vi "Main.vi"(0 "A":dbl=4.0 min=0.0, 5 "B":dbl=2.0, 7 "Calculate":bool, 11 "Error In":errorcluster, 13 "Operation":T1) -> (4 "Output":dbl=6.0, 15 "error out":errorcluster)   [LabVIEW 2021, in "Calculator.lvlib"]
doc: "This VI acts as a simple calculator using OOPS . There are four seperate child classes for each arithmetic operation which has its overriding method operation.vi . The user selects the operation to perform and gives the input. The output is displayed when calculate is pressed."
uses:
  Calculator.lvlib
  Controls/QueueOperations.ctl
  Controls/Operation.ctl
  Controls/DataCluster.ctl
  Classes/NumericOperation/NumericOperation.lvclass
panel:
  in  "Instruction":bool
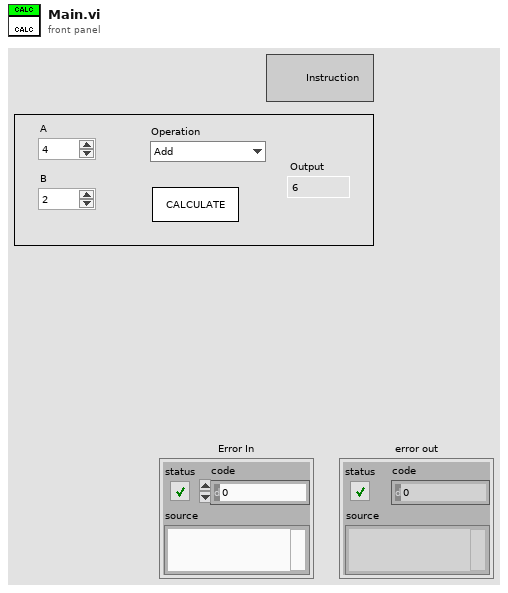
[diagram p1: front panel]
types:
  T1 = typedef "Calculator.lvlib/Operation.ctl" = enum16{"Add", "Subtract", "Multiply", "Divide"}
  T2 = typedef "Calculator.lvlib/QueueOperations.ctl" = enum16{"Create", "Enqueue", "EnqueueN", "Enqueue at Top", "Dequeue", "Flush", "Release"}
  T3 = typedef "Calculator.lvlib/DataCluster.ctl" = cluster{"A":dbl, "B":dbl, "C":dbl, "Operation":T1, "NumericOperation.lvclass":refnum<class "NumericOperation.lvclass">, "generic class reference":refnum<class "NumericOperation.lvclass">, "Base Path":path}
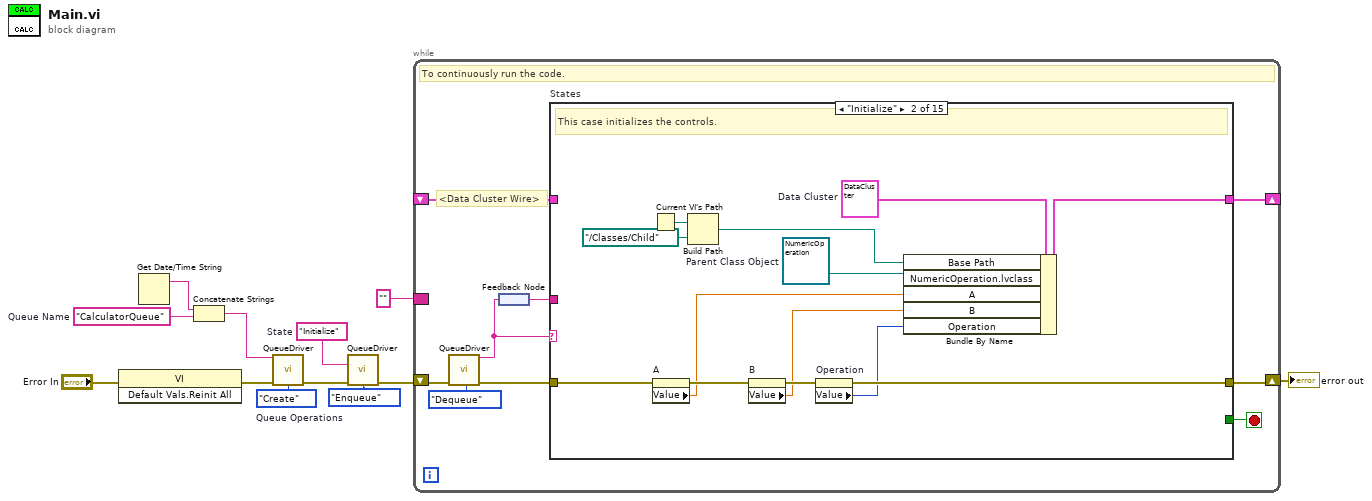
[diagram p0: block diagram]
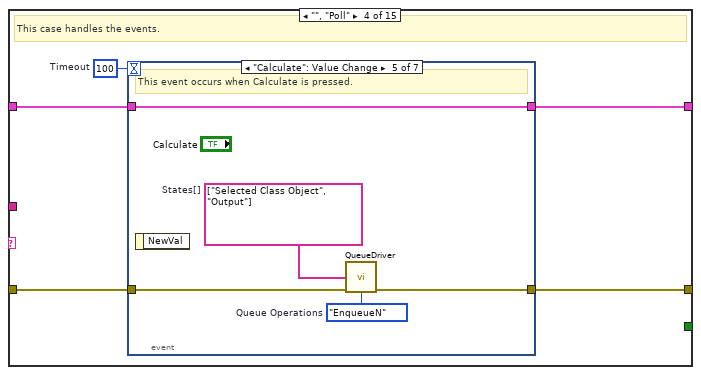
[diagram p4: hidden frame]
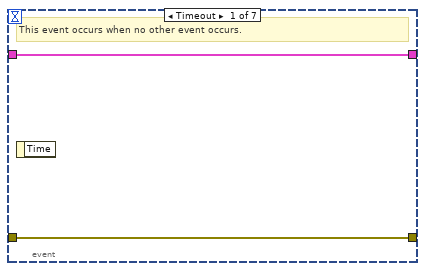
[diagram p5: hidden frame]
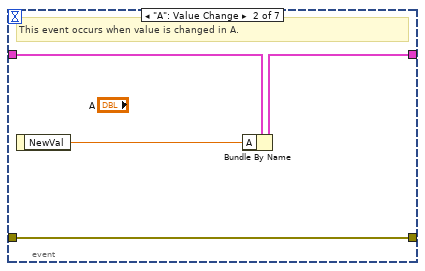
[diagram p6: hidden frame]
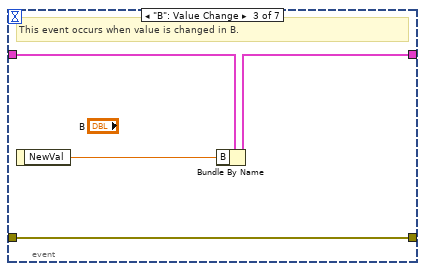
[diagram p7: hidden frame]
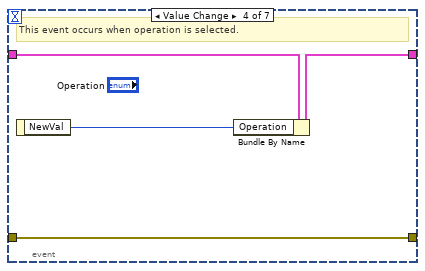
[diagram p8: hidden frame]
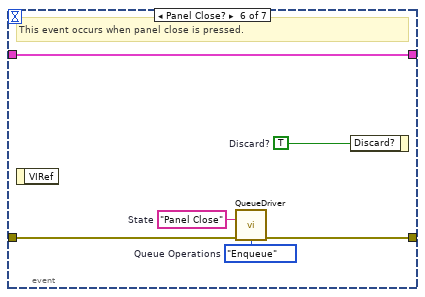
[diagram p9: hidden frame]
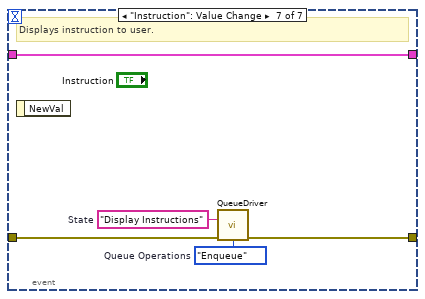
[diagram p10: hidden frame]
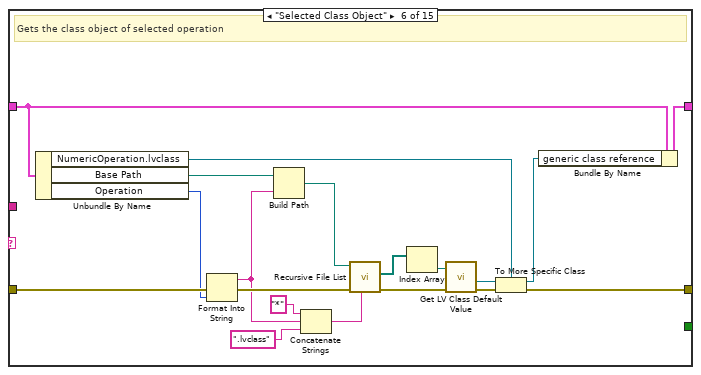
[diagram p12: hidden frame]
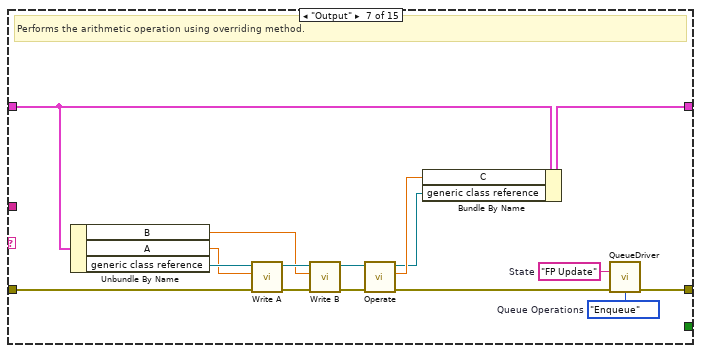
[diagram p13: hidden frame]
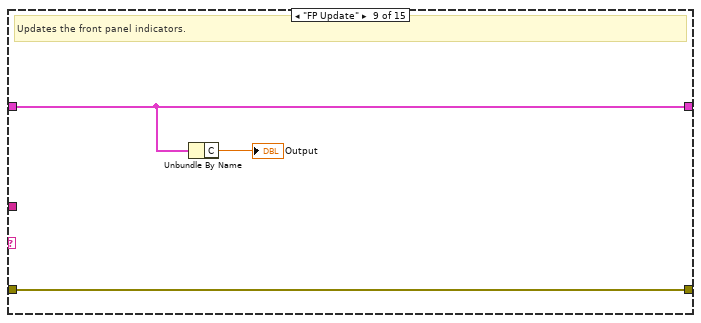
[diagram p15: hidden frame]
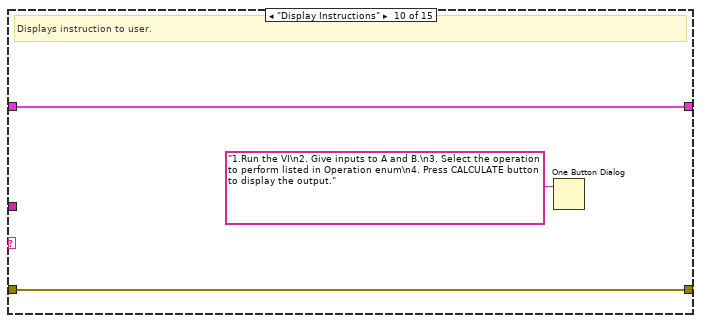
[diagram p16: hidden frame]
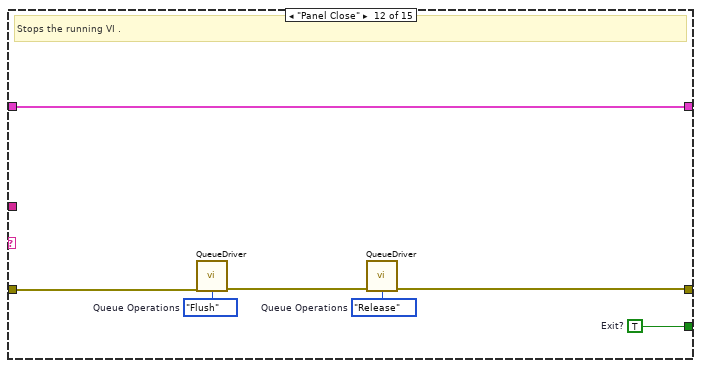
[diagram p18: hidden frame]
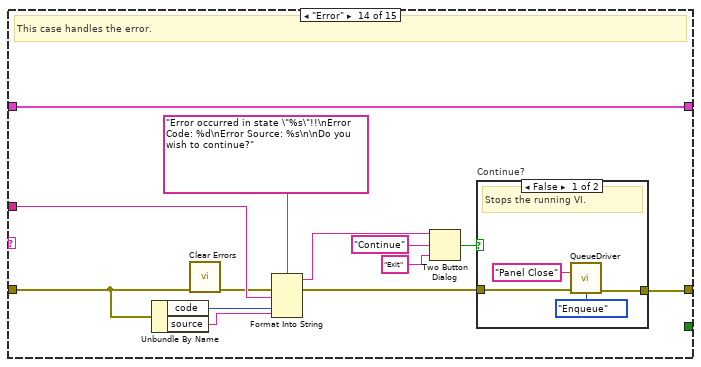
[diagram p20: hidden frame]
diagram:
  w8 = "Initialize"  # State
  w4 = "CalculatorQueue"  # Queue Name
  w11 = QueueOperations."Create"  # Queue Operations
  n1 = invoke class="VI" method="Default Vals.Reinit All"(error in="Error In") -> (error out=w1:errorcluster)  [unwired: 2 in, 2 out]
  n2 = Get Date/Time String() -> (date string=w5:string)  [unwired: 3 in, 1 out]
  n3 = Concatenate Strings(w5, w4) -> (w3:string)
  n4 = call "QueueDriver.vi"("Queue Name"=w3, "Error In"=w1, "Queue Operations"=w11) -> ("Error Out"=w10:errorcluster)  [unwired: 11 in, 1 out]
  n5 = call "QueueDriver.vi"("State"=w8, "Error In"=w10, "Queue Operations"=QueueOperations."Enqueue") -> ("Error Out"=w7:errorcluster)  [unwired: 11 in, 1 out]
  n6 = while {
    shift-right: [w19] -> _
    shift-left: _ -> [w20]
    shift-right: [w17] -> w12
    shift-left: w7 -> [w18]
    border: "" ("Dequeued Element") -> [_]
    stop <- w14 stop-if-true
    # "<Data Cluster Wire>"
    # "To continuously run the code."
    n7 = call "QueueDriver.vi"("Error In"=w18, "Queue Operations"=QueueOperations."Dequeue") -> ("Dequeued Element"=w16:string, "Error Out"=w13:errorcluster)  [unwired: 12 in]
    n8 = feedback-in #1(w16) -> ()
    n9 = feedback #1() -> (w15:string)
    n10 = case "States" shown="\"Initialize\"" w16 {
      tunnel: w20 -> [w23 _ w38 w42 w75 w78 w110 w112 w114 w118 w120 w123 w129 w134 w149]
      tunnel: [w23 w35 w38 w41 w75 w77 w108 w112 w114 w118 w120 w123 w129 w134 w149] -> w19
      tunnel: [w22 w31 w37 w40 w74 w81 w106 w111 w113 w117 w119 w124 w128 w136 w148] -> w17
      tunnel: w15 -> [_ _ _ _ _ _ _ _ _ _ _ _ _ w141 _]
      tunnel: [_ _ _ _ _ _ _ _ _ _ _ w122 _ _ _] -> w14
      tunnel: w13 -> [w22 w34 w37 w39 w74 w94 w96 w111 w113 w117 w119 w121 w128 w131 w148]
      frame "/******** Initialize********/" {
        # "Splitter case for initialization."
      }
      frame "Initialize" {
        w27 = T3 {"A"=0.0, "B"=0.0, "C"=0.0, "Operation"=enum."Add", "NumericOperation.lvclass"=refnum, "generic class reference"=refnum, "Base Path"=path ""}  # Data Cluster
        w36 = refnum<class "NumericOperation.lvclass"> refnum  # Parent Class Object
        # "This case initializes the controls."
        n11 = Current VI's Path() -> (path=w26:path)
        n12 = property on="A" class="DigNum (strict)"(error in=w34) -> (error out=w33:errorcluster, "Value"=w28:dbl)  [unwired: 1 in, 1 out]
        n13 = Build Path(base path=w26, name or relative path=path "../Classes/Child") -> (appended path=w24:path)
        n14 = property on="B" class="DigNum (strict)"(error in=w33) -> (error out=w32:errorcluster, "Value"=w29:dbl)  [unwired: 1 in, 1 out]
        n15 = property on="Operation" class="Enum (strict)"(error in=w32) -> (error out=w31:errorcluster, "Value"=w30:T1)  [unwired: 1 in, 1 out]
        n16 = Bundle By Name(cluster=w27, "Base Path"=w24, "NumericOperation.lvclass"=w36, "A"=w28, "B"=w29, "Operation"=w30) -> (w35:T3)
      }
      frame "/******** Poll ********/" {
        # "Splitter case for poll."
      }
      frame "", "Poll" {
        w43 = 100  # Timeout
        # "This case handles the events."
        n17 = event shown="[4] \"Calculate\": Value Change" {
          selector: _ -> [_ _ _ _ _ _ _]
          dyn-events: _ -> [_ _ _ _ _ _ _]
          timeout: w43 -> [_ _ _ _ _ _ _]
          tunnel: w42 -> [w45 w49 w53 w57 w62 w65 w69]
          tunnel: [w45 w47 w51 w55 w62 w65 w69] -> w41
          tunnel: [w44 w46 w50 w54 w60 w67 w72] -> w40
          tunnel: w39 -> [w44 w46 w50 w54 w61 w63 w73]
          event Timeout {
            # "This event occurs when no other event occurs."
            n18 = event-data() -> ()  [unwired: 1 in, 1 out]
          }
          event "A": Value Change {
            # "This event occurs when value is changed in A."
            n19 = event-data() -> ("NewVal"=w48:dbl)  [unwired: 1 in]
            n20 = Bundle By Name(cluster=w49, "A"=w48) -> (w47:T3)
          }
          event "B": Value Change {
            # "This event occurs when value is changed in B."
            n21 = event-data() -> ("NewVal"=w52:dbl)  [unwired: 1 in]
            n22 = Bundle By Name(cluster=w53, "B"=w52) -> (w51:T3)
          }
          event Value Change {
            # "This event occurs when operation is selected."
            n23 = event-data() -> ("NewVal"=w56:T1)  [unwired: 1 in]
            n24 = Bundle By Name(cluster=w57, "Operation"=w56) -> (w55:T3)
          }
          event "Calculate": Value Change {
            w58 = string[] ["Selected Class Object", "Output"]  # States[]
            w59 = QueueOperations."EnqueueN"  # Queue Operations
            # "This event occurs when Calculate is pressed."
            n25 = event-data() -> ()  [unwired: 1 in, 1 out]
            n26 = call "QueueDriver.vi"("States[]"=w58, "Error In"=w61, "Queue Operations"=w59) -> ("Error Out"=w60:errorcluster)  [unwired: 11 in, 1 out]
          }
          event Panel Close? {
            w64 = QueueOperations."Enqueue"  # Queue Operations
            w66 = "Panel Close"  # State
            w68 = TRUE  # Discard?
            # "This event occurs when panel close is pressed."
            n27 = event-data() -> ()  [unwired: 1 in, 1 out]
            n28 = call "QueueDriver.vi"("State"=w66, "Error In"=w63, "Queue Operations"=w64) -> ("Error Out"=w67:errorcluster)  [unwired: 11 in, 1 out]
            n29 = event-data("Discard?"=w68) -> ()  [unwired: 1 in, 1 out]
          }
          event "Instruction": Value Change {
            w70 = "Display Instructions"  # State
            w71 = QueueOperations."Enqueue"  # Queue Operations
            # "Displays instruction to user."
            n30 = event-data() -> ()  [unwired: 1 in, 1 out]
            n31 = call "QueueDriver.vi"("State"=w70, "Error In"=w73, "Queue Operations"=w71) -> ("Error Out"=w72:errorcluster)  [unwired: 11 in, 1 out]
          }
        }
      }
      frame "/******** Functionalities ********/" {
        # "Splitter case for functionalities."
      }
      frame "Selected Class Object" {
        # "Gets the class object of selected operation"
        n32 = Unbundle By Name(w78) -> ("NumericOperation.lvclass"=w79:refnum<class "NumericOperation.lvclass">, "Base Path"=w92:path, "Operation"=w93:T1)
        n33 = Format Into String(error in=w94, w93) -> (resulting string=w88:string, error out=w91:errorcluster)  [unwired: 2 in]
        n34 = Build Path(base path=w92, name or relative path=w88) -> (appended path=w90:path)
        n35 = Concatenate Strings("*" ("string"), w88, ".lvclass" ("string")) -> (w86:string)
        n36 = call <vilib>:"Recursive File List.vi"("pattern"=w86, "error in (no error)"=w91, "Folder Path"=w90) -> ("error out"=w84:errorcluster, "All Files in Dir"=w85:path[])  [unwired: 4 in, 3 out]
        n37 = Index Array(array=w85) -> (element=w83:path)  [unwired: 1 in]
        n38 = call <vilib>:"Get LV Class Default Value.vi"("error in (no error)"=w84, "class path"=w83) -> ("error out"=w82:errorcluster, "object"=w80:refnum<class>)  [unwired: 8 in]
        n39 = To More Specific Class(target class=w79, reference=w80, error in=w82) -> (specific class reference=w76:refnum<class "NumericOperation.lvclass">, error out=w81:errorcluster)
        n40 = Bundle By Name(cluster=w78, "generic class reference"=w76) -> (w77:T3)
      }
      frame "Output" {
        w104 = "FP Update"  # State
        w105 = QueueOperations."Enqueue"  # Queue Operations
        # "Performs the arithmetic operation using overriding method."
        n41 = Unbundle By Name(w110) -> ("B"=w97:dbl, "A"=w98:dbl, "generic class reference"=w101:refnum<class "NumericOperation.lvclass">)
        n42 = call-dynamic "Write A.vi"("error in (no error)"=w96, "A"=w98, "NumericOperation in"=w101) -> ("error out"=w103:errorcluster, "NumericOperation out"=w100:refnum<class "NumericOperation.lvclass">)  [unwired: 7 in]
        n43 = call-dynamic "Write B.vi"("error in (no error)"=w103, "B"=w97, "NumericOperation in"=w100) -> ("error out"=w102:errorcluster, "NumericOperation out"=w99:refnum<class "NumericOperation.lvclass">)  [unwired: 7 in]
        n44 = call-dynamic "Operate.vi"("error in (no error)"=w102, "NumericOperation in"=w99) -> ("error out"=w107:errorcluster, "C"=w109:dbl, "NumericOperation out"=w95:refnum<class "NumericOperation.lvclass">)  [unwired: 7 in]
        n45 = Bundle By Name(cluster=w110, "C"=w109, "generic class reference"=w95) -> (w108:T3)
        n46 = call "QueueDriver.vi"("State"=w104, "Error In"=w107, "Queue Operations"=w105) -> ("Error Out"=w106:errorcluster)  [unwired: 11 in, 1 out]
      }
      frame "/******** Front Panel Updates ********/" {
        # "Splitter case for front panel updates."
      }
      frame "FP Update" {
        # "Updates the front panel indicators."
        n47 = Unbundle By Name(w114) -> ("C"=→"Output":dbl)
      }
      frame "Display Instructions" {
        # "Displays instruction to user."
        n48 = One Button Dialog(message="1.Run the VI\n2. Give inputs to A and B.\n3. Select the operation to perform listed in Operation enum\n4. Press CALCULATE button to display the output.") -> ()  [unwired: 1 in, 1 out]
      }
      frame "/******** Panel Close ********/" {
        # "Splitter case for stoping the running VI."
      }
      frame "Panel Close" {
        w122 = TRUE  # Exit?
        w126 = QueueOperations."Release"  # Queue Operations
        w127 = QueueOperations."Flush"  # Queue Operations
        # "Stops the running VI ."
        n49 = call "QueueDriver.vi"("Error In"=w121, "Queue Operations"=w127) -> ("Error Out"=w125:errorcluster)  [unwired: 12 in, 1 out]
        n50 = call "QueueDriver.vi"("Error In"=w125, "Queue Operations"=w126) -> ("Error Out"=w124:errorcluster)  [unwired: 12 in, 1 out]
      }
      frame "/******** Error handling ********/" {
        # "Splitter case for error handling."
      }
      frame "Error" {
        # "This case handles the error."
        n51 = Unbundle By Name(w131) -> ("code"=w132:i32, "source"=w130:string)
        n52 = call <vilib>:"Clear Errors.vi"("error in (no error)"=w131) -> ("error out"=w133:errorcluster)  [unwired: 5 in, 1 out]
        n53 = Format Into String(format string="Error occurred in state \"%s\"!!\nError Code: %d\nError Source: %s\n\nDo you wish to continue?", error in=w133, w141, w132, w130) -> (resulting string=w138:string, error out=w137:errorcluster)  [unwired: 1 in]
        n54 = Two Button Dialog(message=w138, 1:"Exit" ("F button name (\"Cancel\")"), 2:"Continue" ("T button name (\"OK\")")) -> (T button?=w135:bool)
        n55 = case "Continue?" shown="False" w135 {
          tunnel: w137 -> [w146 w147]
          tunnel: [w145 w147] -> w136
          frame False {
            # "Stops the running VI."
            n56 = call "QueueDriver.vi"("State"="Panel Close", "Error In"=w146, "Queue Operations"=QueueOperations."Enqueue") -> ("Error Out"=w145:errorcluster)  [unwired: 11 in, 1 out]
          }
          frame True {
            # "Continue"
          }
        }
      }
      frame Default {
        # "This case handles the developer error."
      }
    }
  }
  "error out" <- w12
